vi "SEK2020v1AndarReto.vi"(1 "NXT/EV3":T1) -> (8 "NXT/EV3 2":T1)   [LabVIEW 2016]
uses:
  <vilib>/NXT/Subs/LVHSConnector.ctl
  <vilib>/NXT/LegoClasses/BrickReference/BrickReference.lvclass
  <vilib>/NXT/Block Support/NXT_InputPort.ctl
  <vilib>/NXT/Block Support/NXT_OutputPort.ctl
  <vilib>/NXT/Dual Mode Library/Sensors/EV3_Gyro_Angle.vi
  <vilib>/NXT/NXTIO Xnodes/NXTIONodeSubVIs/NXTMoveMotors.vi
  <vilib>/NXT/NXTIO Xnodes/AddressXNode/NXTIOAddress.xnode
  <vilib>/NXT/NXTIO Xnodes/NXTIOXNode/NXTIO.xnode
panel:
  in  "Kd":sgl
  in  "Ki":sgl
  in  "Kp":sgl=2.0
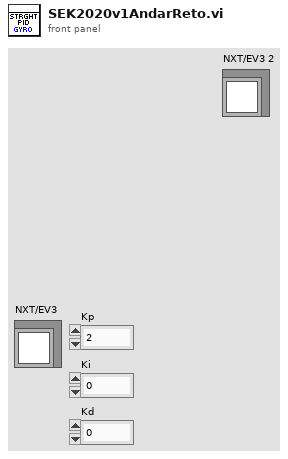
[diagram p1: front panel]
types:
  T1 = typedef "LVHSConnector.ctl" = refnum<class "BrickReference.lvclass">
  T2 = typedef "NXT_InputPort.ctl" = u32
  T3 = typedef "NXT_OutputPort.ctl" = u8
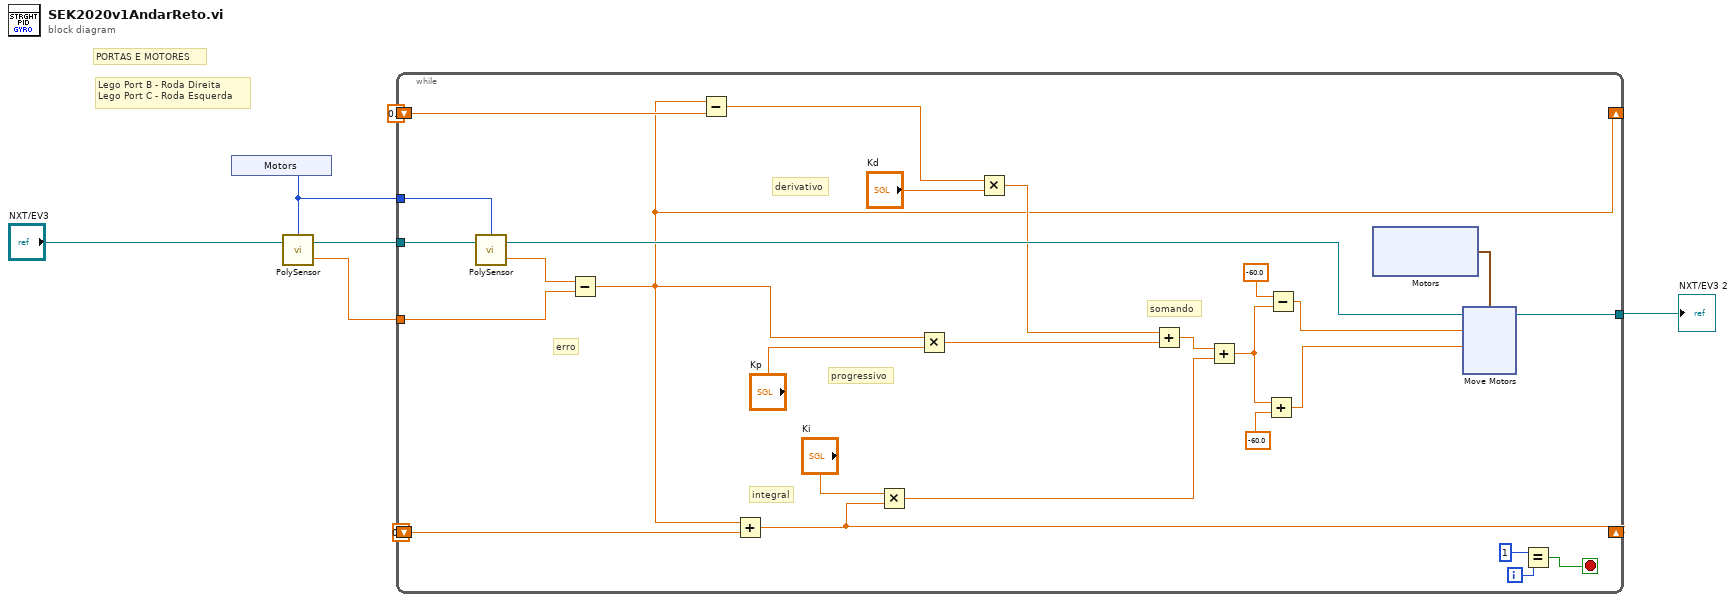
[diagram p0: block diagram]
diagram:
  # "Lego Port B - Roda Direita\nLego Port C - Roda Esquerda"
  # "PORTAS E MOTORES"
  n1 = xnode "Motors"() -> ("Sensor"=w2:T2)
  n2 = call-poly <vilib>:"PolySensor.vi"("NXT/EV3"="NXT/EV3", "Port (Port 1)"=w2) -> ("Degrees"=w1:sgl, "NXT/EV3"=w7:T1)  [unwired: 1 in]
  n3 = while {
    tunnel: w7 -> [w34]
    shift-right: [w21] -> _
    shift-left: sgl 0.0 -> [w23]
    shift-right: [w16] -> _
    shift-left: sgl 0.0 -> [w18]
    tunnel: w2 -> [w13]
    tunnel: [w11] -> w4
    tunnel: w1 -> [w12]
    i -> [w10]
    stop <- w8 stop-if-true
    # "somando"
    # "erro"
    # "progressivo"
    # "integral"
    # "derivativo"
    n4 = call-poly <vilib>:"PolySensor.vi"("NXT/EV3"=w34, "Port (Port 1)"=w13) -> ("Degrees"=w17:sgl, "NXT/EV3"=w24:T1)  [unwired: 1 in]
    n5 = Subtract(x=w17, y=w12) -> (x-y=w16:sgl)
    n6 = Subtract(x=w16, y=w18) -> (x-y=w14:sgl)
    n7 = Add(x=w16, y=w23) -> (x+y=w21:sgl)
    n8 = Multiply(x="Ki", y=w21) -> (x*y=w20:sgl)
    n9 = Multiply(x=w16, y="Kp") -> (x*y=w27:sgl)
    n10 = Multiply(x=w14, y="Kd") -> (x*y=w19:sgl)
    n11 = Add(x=w19, y=w27) -> (x+y=w25:sgl)
    n12 = Add(x=w25, y=w20) -> (x+y=w26:sgl)
    n13 = Add(x=w26, y=sgl -60.0) -> (x+y=w28:sgl)
    n14 = Subtract(x=sgl -60.0, y=w26) -> (x-y=w31:sgl)
    n15 = xnode "Motors"() -> ("Motor"=w33:cluster{"Port":T3, "Port":T3})
    n16 = xnode "Move Motors"("Power/Speed 2"=w28, "Power/Speed 1"=w31, "Motors"=w33, "NXT/EV3"=w24) -> ("NXT/EV3"=w11:T1)
    n17 = Equal?(x=1, y=w10) -> (x = y?=w8:bool)
  }
  "NXT/EV3 2" <- w4
